vi "Initialize Custom Device.vi"(8 "error in":errorcluster, 11 "Item Ref in":u64 format="%.0x") -> (0 "error out":errorcluster, 3 "Item Ref out":u64=18446744073709551615 format="%.0x")   [LabVIEW 2026, in "NIDMM Configuration.lvlib"]
uses:
  NIDMM Configuration.lvlib
  NationalInstruments.VeriStand.SystemDefinitionAPI
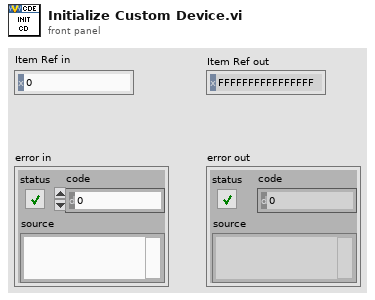
[diagram p1: front panel]
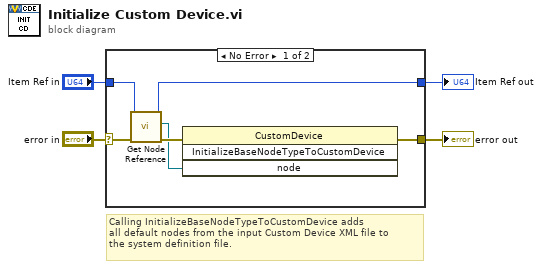
[diagram p0: block diagram]
diagram:
  # "Calling InitializeBaseNodeTypeToCustomDevice adds \nall default nodes from the input Custom Device XML file to \nthe system definition file."
  n1 = case shown="No Error" "error in" {
    selector: "error in" -> [w10 w12]
    tunnel: "Item Ref in" -> [w9 w11]
    tunnel: [w8 w11] -> w2
    tunnel: [w6 w12] -> w1
    frame No Error {
      n2 = call "Get Node Reference.vi"("error in"=w10, "Item Ref in"=w9) -> ("error out"=w7:errorcluster, "Base Node Type"=w5:refnum<k24>, "Item Ref out"=w8:u64)  [unwired: 6 in, 1 out]
      n3 = invoke class="CustomDevice" method="InitializeBaseNodeTypeToCustomDevice"(error in=w7, "node"=w5) -> (error out=w6:errorcluster)  [unwired: 2 in, 3 out]
    }
    frame Error {
    }
  }
  "error out" <- w1
  "Item Ref out" <- w2
